vi "Get Room Info.vi"(8 "error in (no error)":errorcluster, 10 "Room GUID":string, 11 "Room-API in":refnum<class "Room-API.lvclass">) -> (0 "error out":errorcluster, 1 "Room Info":T1, 2 "found?":bool, 3 "Room-API out":refnum<class "Room-API.lvclass">)   [LabVIEW 2020, in "Room-API.lvclass"]
uses:
  Room-API.lvclass
  Single Room.ctl
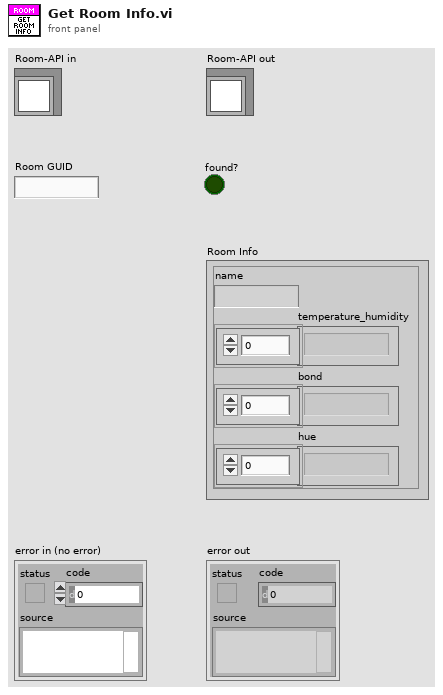
[diagram p1: front panel]
types:
  T1 = typedef "Room-API.lvclass/Single Room.ctl" = cluster{"name":string, "temperature_humidity":string[], "bond":string[], "hue":string[]}
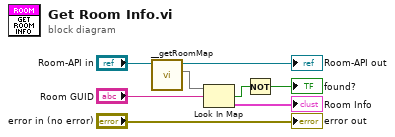
[diagram p0: block diagram]
diagram:
  n1 = call "__getRoomMap.vi"("Room-API in"="Room-API in") -> ("room_map"=w6:map{string, T1}, "Room-API out"=→"Room-API out":refnum<class "Room-API.lvclass">)  [unwired: 9 in]
  n2 = Look In Map(map=w6, key="Room GUID") -> (key not found?=w3:bool, value=→"Room Info":T1)  [unwired: 1 in]
  n3 = Not(x=w3) -> (.not. x?=→"found?":bool)
  "error out" <- "error in (no error)"
